vi "CLD1015.vi"() -> ()   [LabVIEW 2021]
uses:
  <vilib>/Analysis/baseanly.llb/Mean (DBL).vi
  <vilib>/Analysis/NI_AALBase.lvlib
panel:
  in  "Iteration":u64
  in  "Steps":u64
  in  "Stop":dbl
  in  "Start":dbl
  out "Horizontal Pointer Slide":dbl(slide) scale=0.0..100.0
  out "Averaged":cluster{"X":dbl, "Y":dbl}[](graph)
  out "Single shot":cluster{"X":dbl, "Y":dbl}[](graph)
  in  "Set current":bool
  out "Temperature":dbl(graph)
  out "Laser Current":dbl(graph)
  in  "Modulation":bool
  in  "Temperature Unit":i16(ring) caption="Temperature Unit (Degrees Celsius)" items=["Degrees Celsius", "Kelvin", "Degrees Fahrenheit"]
  in  "Disp. Auto-Dim.":bool
  in  "Disp. Brightness":dbl min=0.0 max=1.0 step=0.1
  in  "Send Utility\nSettings":bool
  in  "Send LD/TEC\nSettings":bool
  in  "Temperature Set":dbl=15.0 caption="Temperature" min=15.0 max=45.0 step=0.5
  in  "Laser Current Set":dbl caption="Laser Current" min=0.0 max=0.145 step=0.005
  out "Photodiode Current":dbl caption="Photodiode Current (0)"
  out "Thermopile Voltage":dbl caption="Thermopile Voltage (0)"
  out "Power":dbl caption="Power (0)"
  out "Laser Voltage":dbl caption="Laser Voltage (0)"
  out "Laser Current":dbl
  out "Optical Power Pd":dbl caption="Optical Power Pd (0)"
  out "Optical Power Th":dbl caption="Optical Power Th (0)"
  out "Temperature":dbl
  in  "Turn Off Program":bool
  in  "TEC Switch":bool
  in  "LD Switch":bool
  out "TEC Setpoint High Limit":dbl caption="Setpoint High Limit"
  out "TEC Setpoint Low Limit":dbl caption="Setpoint Low Limit"
  out "TEC Operating Mode":enum16{"Current", "Temperature"}(ring)
  out "LD Current Limit":dbl caption="Laser Diode Current Limit"
  in  "resource name":refnum<visa-resource-name>="Probe_laser"
  # "For the program to work properly one have to connect SAS signal to AI7\n and CLD1015 modulation channel to AO0"
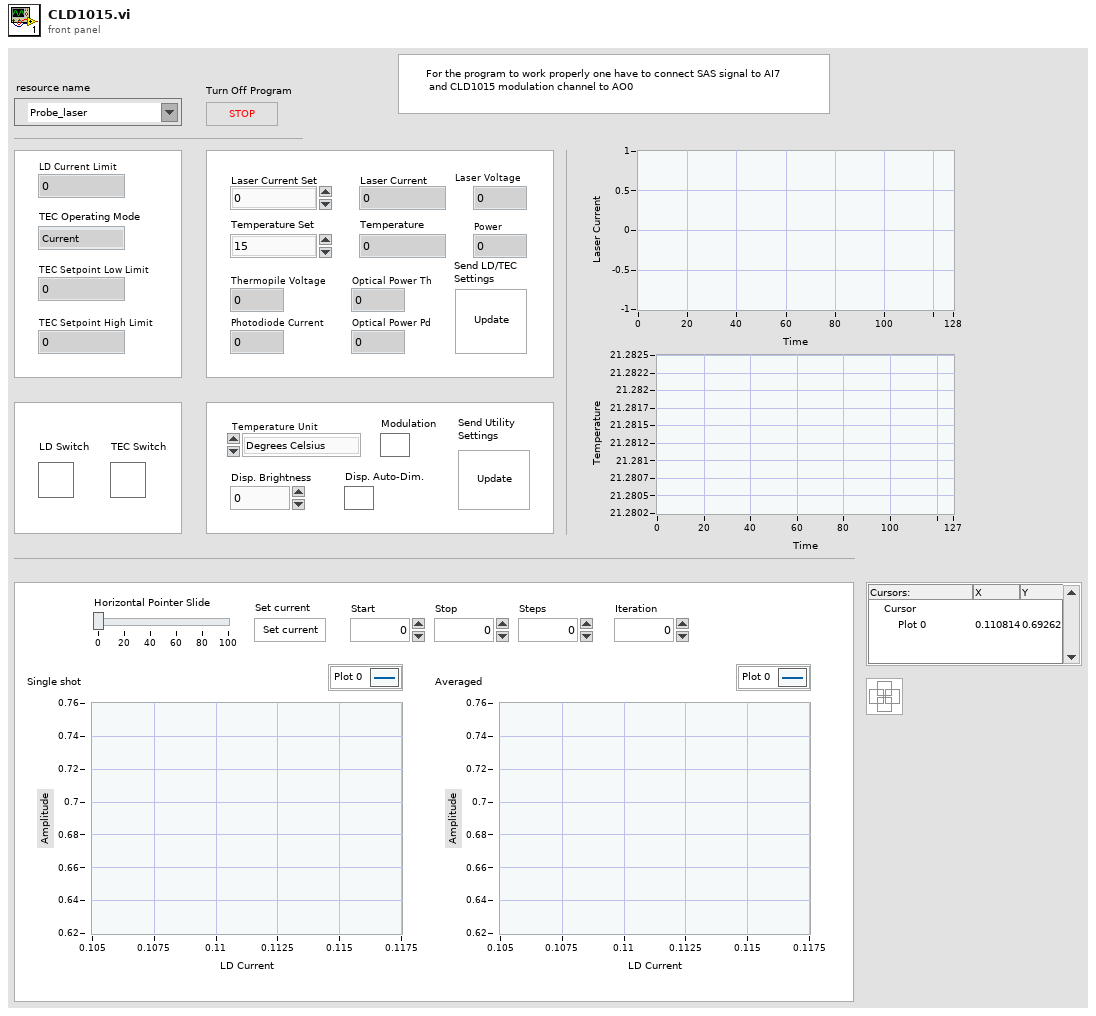
[diagram p1: front panel]
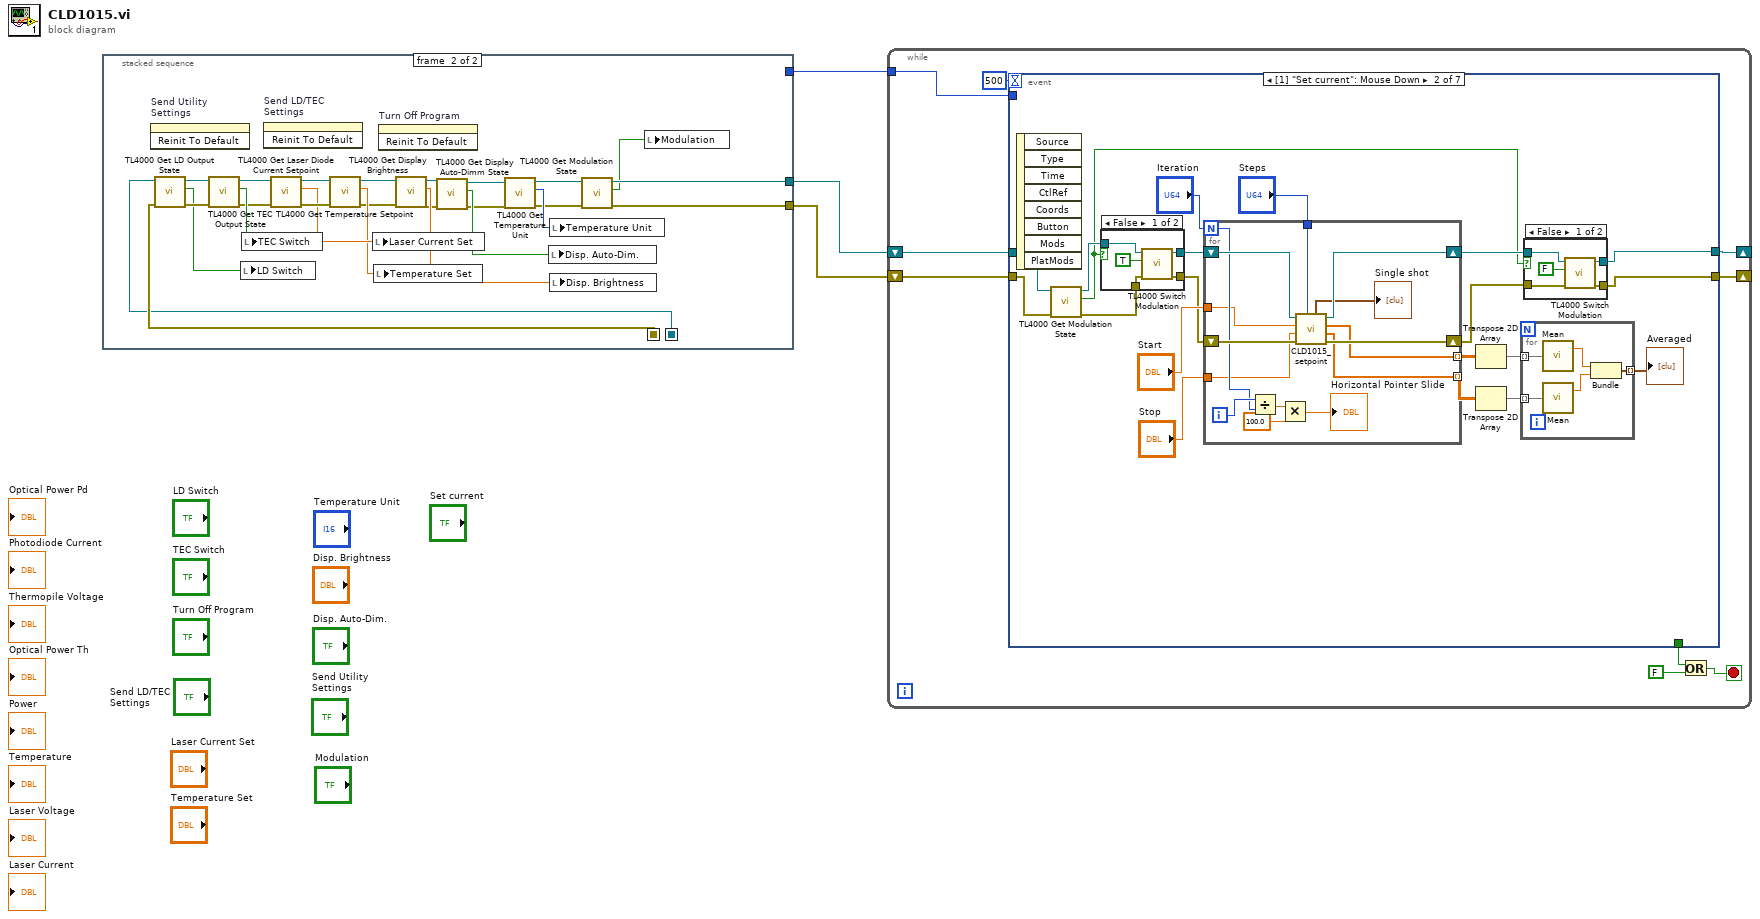
[diagram p0: block diagram]
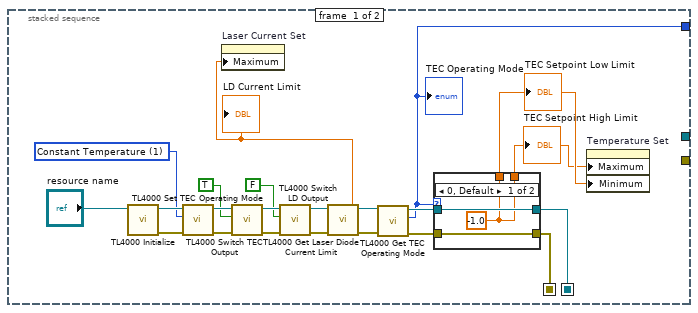
[diagram p2: hidden frame]
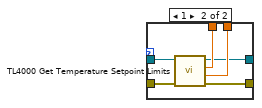
[diagram p3: hidden frame]
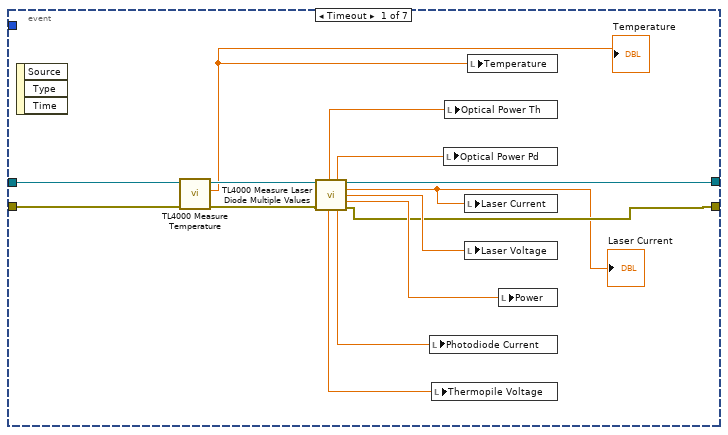
[diagram p4: hidden frame]
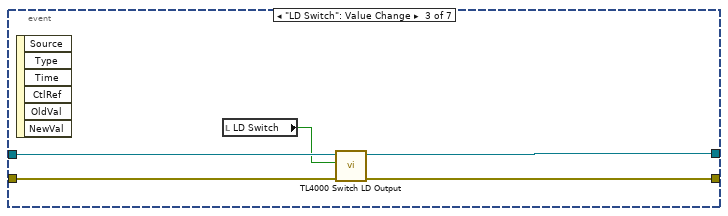
[diagram p7: hidden frame]
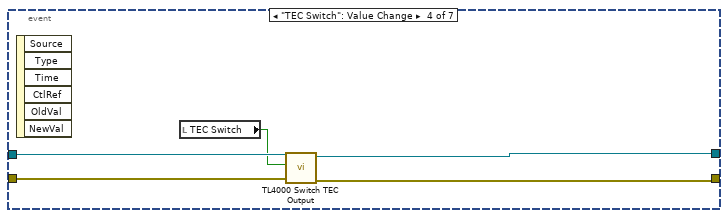
[diagram p8: hidden frame]
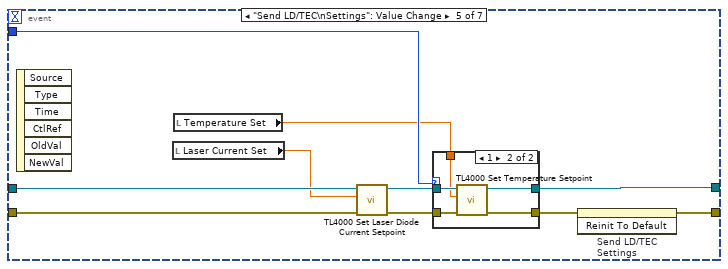
[diagram p9: hidden frame]
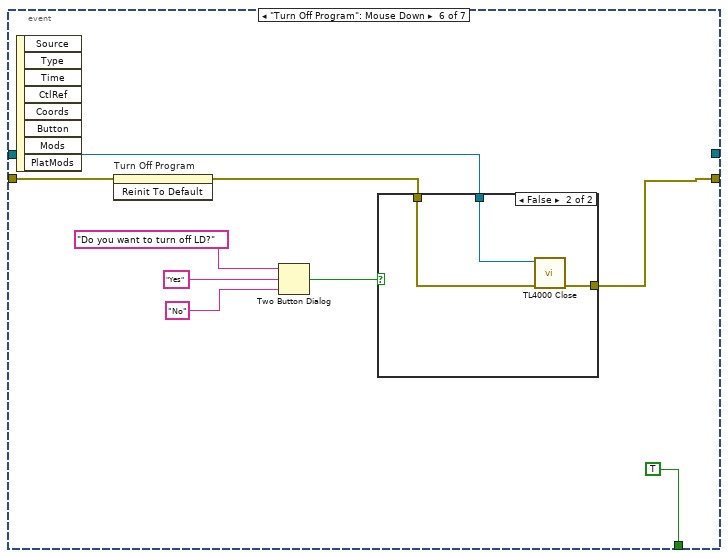
[diagram p11: hidden frame]
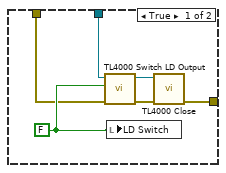
[diagram p12: hidden frame]
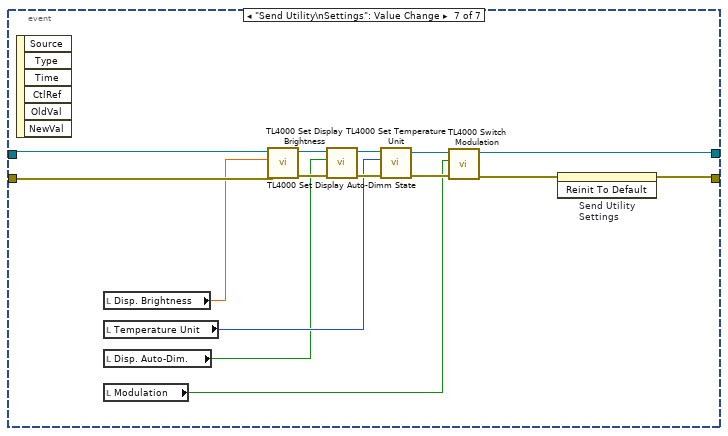
[diagram p13: hidden frame]
diagram:
  n1 = stacked-sequence {
    seq-local: [w9 _] -> [_ w57]
    seq-local: [w8 _] -> [_ w58]
    tunnel: [_ w36] -> w2
    tunnel: [_ w37] -> w1
    tunnel: [w7 _] -> w3
    frame #0 {
      w22 = i16 1 items=["Constant Temperature"=1, "Current Source"=0] ("TEC Operating Mode (Constant Temperature)")
      n2 = call <instrlib>:"TL4000 Initialize.vi"("resource name"="resource name") -> ("error out"=w24:errorcluster, "instrument handle out"=w23:refnum<visa-resource-name>)  [unwired: 9 in]
      n3 = call <instrlib>:"TL4000 Set TEC Operating Mode.vi"("error in (no error)"=w24, "TEC Operating Mode (Constant Temperature)"=w22, "instrument handle"=w23) -> ("error out"=w21:errorcluster, "instrument handle out"=w20:refnum<visa-resource-name>)  [unwired: 7 in]
      n4 = call <instrlib>:"TL4000 Switch TEC Output.vi"("error in (no error)"=w21, "TEC Output (Off)"=TRUE, "instrument handle"=w20) -> ("error out"=w18:errorcluster, "instrument handle out"=w17:refnum<visa-resource-name>)  [unwired: 7 in]
      n5 = call <instrlib>:"TL4000 Switch LD Output.vi"("error in (no error)"=w18, "LD Output (Off)"=FALSE, "instrument handle"=w17) -> ("error out"=w15:errorcluster, "instrument handle out"=w14:refnum<visa-resource-name>)  [unwired: 7 in]
      n6 = call <instrlib>:"TL4000 Get Laser Diode Current Limit.vi"("error in (no error)"=w15, "instrument handle"=w14) -> ("error out"=w13:errorcluster, "Laser Diode Current Limit"=w6:dbl, "instrument handle out"=w12:refnum<visa-resource-name>)  [unwired: 7 in]
      "LD Current Limit" <- w6
      n7 = property on="Laser Current Set" class="DigNum (strict)"("Maximum"=w6) -> ()  [unwired: 2 in, 2 out]
      n8 = call <instrlib>:"TL4000 Get TEC Operating Mode.vi"("error in (no error)"=w13, "instrument handle"=w12) -> ("error out"=w10:errorcluster, "TEC Operating Mode"=w7:i16, "instrument handle out"=w11:refnum<visa-resource-name>)  [unwired: 7 in]
      "TEC Operating Mode" <- w7
      n9 = case shown="0, Default" w7 {
        tunnel: w11 -> [w28 w33]
        tunnel: w10 -> [w27 w34]
        tunnel: [w26 w32] -> w5
        tunnel: [w26 w31] -> w4
        tunnel: [w28 w30] -> w9
        tunnel: [w27 w29] -> w8
        frame 0, Default {
          w26 = -1.0
        }
        frame 1 {
          n10 = call <instrlib>:"TL4000 Get Temperature Setpoint Limits.vi"("error in (no error)"=w34, "instrument handle"=w33) -> ("error out"=w29:errorcluster, "Setpoint High Limit"=w31:dbl, "Setpoint Low Limit"=w32:dbl, "instrument handle out"=w30:refnum<visa-resource-name>)  [unwired: 6 in]
        }
      }
      "TEC Setpoint Low Limit" <- w5
      "TEC Setpoint High Limit" <- w4
      n11 = property on="Temperature Set" class="DigNum (strict)"("Maximum"=w4, "Minimum"=w5) -> ()  [unwired: 2 in, 2 out]
    }
    frame #1 {
      n12 = invoke on="Send Utility\nSettings" class="Bool (strict)" method="Reinit To Default"() -> ()  [unwired: 3 in, 3 out]
      n13 = call <instrlib>:"TL4000 Get LD Output State.vi"("error in (no error)"=w58, "instrument handle"=w57) -> ("error out"=w59:errorcluster, "LD Output"=w56:bool, "instrument handle out"=w60:refnum<visa-resource-name>)  [unwired: 7 in]
      n14 = call <instrlib>:"TL4000 Get TEC Output State.vi"("error in (no error)"=w59, "instrument handle"=w60) -> ("error out"=w53:errorcluster, "TEC Output"=w55:bool, "instrument handle out"=w54:refnum<visa-resource-name>)  [unwired: 7 in]
      n15 = local write "LD Switch"(w56) -> ()
      n16 = local write "TEC Switch"(w55) -> ()
      n17 = invoke on="Send LD/TEC\nSettings" class="Bool (strict)" method="Reinit To Default"() -> ()  [unwired: 3 in, 3 out]
      n18 = call <instrlib>:"TL4000 Get Laser Diode Current Setpoint.vi"("error in (no error)"=w53, "instrument handle"=w54) -> ("error out"=w51:errorcluster, "Laser Diode Current Setpoint"=w50:dbl, "instrument handle out"=w52:refnum<visa-resource-name>)  [unwired: 7 in]
      n19 = call <instrlib>:"TL4000 Get Temperature Setpoint.vi"("error in (no error)"=w51, "instrument handle"=w52) -> ("error out"=w40:errorcluster, "Temperature Setpoint"=w49:dbl, "instrument handle out"=w41:refnum<visa-resource-name>)  [unwired: 7 in]
      n20 = local write "Laser Current Set"(w50) -> ()
      n21 = local write "Temperature Set"(w49) -> ()
      n22 = invoke on="Turn Off Program" class="Bool" method="Reinit To Default"() -> ()  [unwired: 3 in, 3 out]
      n23 = call <instrlib>:"TL4000 Get Display Brightness.vi"("error in (no error)"=w40, "instrument handle"=w41) -> ("error out"=w45:errorcluster, "Brightness"=w46:dbl, "instrument handle out"=w42:refnum<visa-resource-name>)  [unwired: 7 in]
      n24 = call <instrlib>:"TL4000 Get Display Auto-Dimm State.vi"("error in (no error)"=w45, "instrument handle"=w42) -> ("error out"=w44:errorcluster, "Auto-Dimm State"=w47:bool, "instrument handle out"=w43:refnum<visa-resource-name>)  [unwired: 7 in]
      n25 = call <instrlib>:"TL4000 Get Temperature Unit.vi"("error in (no error)"=w44, "instrument handle"=w43) -> ("error out"=w38:errorcluster, "Temperature Unit"=w48:i16, "instrument handle out"=w39:refnum<visa-resource-name>)  [unwired: 7 in]
      n26 = local write "Disp. Auto-Dim."(w47) -> ()
      n27 = local write "Temperature Unit"(w48) -> ()
      n28 = local write "Disp. Brightness"(w46) -> ()
      n29 = call <instrlib>:"TL4000 Get Modulation State.vi"("error in (no error)"=w38, "instrument handle"=w39) -> ("error out"=w37:errorcluster, "Modulation State"=w35:bool, "instrument handle out"=w36:refnum<visa-resource-name>)  [unwired: 7 in]
      n30 = local write "Modulation"(w35) -> ()
    }
  }
  n31 = while {
    shift-right: [w68] -> _
    shift-left: w1 -> [w69]
    tunnel: w3 -> [w62]
    shift-right: [w67] -> _
    shift-left: w2 -> [w61]
    stop <- w66 stop-if-true
    n32 = event shown="[1] \"Set current\": Mouse Down" {
      selector: _ -> [_ _ _ _ _ _ _]
      dyn-events: _ -> [_ _ _ _ _ _ _]
      timeout: 500 -> [_ _ _ _ _ _ _]
      tunnel: w61 -> [w83 w94 w142 w147 w157 w166 w193]
      tunnel: w69 -> [w82 w93 w141 w146 w148 w172 w192]
      tunnel: [w72 w85 w139 w144 w149 w165 w188] -> w68
      tunnel: [w73 w86 w138 w145 w151 _ w185] -> w67
      tunnel: [_ _ _ _ _ TRUE _] -> w64
      tunnel: w62 -> [_ _ _ _ w155 _ _]
      event Timeout {
        n33 = event-data() -> ()  [unwired: 1 in, 3 out]
        n34 = call <instrlib>:"TL4000 Measure Temperature.vi"("error in (no error)"=w82, "instrument handle"=w83) -> ("error out"=w80:errorcluster, "Temperature"=w71:dbl, "instrument handle out"=w81:refnum<visa-resource-name>)  [unwired: 7 in]
        "Temperature" <- w71
        n35 = call <instrlib>:"TL4000 Measure Laser Diode Multiple Values.vi"("instrument handle"=w81, "error in (no error)"=w80) -> ("Optical Power Th (0)"=w79:dbl, "Optical Power Pd (0)"=w78:dbl, "instrument handle out"=w73:refnum<visa-resource-name>, "Laser Current"=w70:dbl, "Laser Voltage (0)"=w77:dbl, "Power (0)"=w76:dbl, "Thermopile Voltage (0)"=w75:dbl, "Photodiode Current (0)"=w74:dbl, "error out"=w72:errorcluster)  [unwired: 5 in]
        "Laser Current" <- w70
        n36 = local write "Photodiode Current"(w74) -> ()
        n37 = local write "Thermopile Voltage"(w75) -> ()
        n38 = local write "Optical Power Pd"(w78) -> ()
        n39 = local write "Optical Power Th"(w79) -> ()
        n40 = local write "Laser Current"(w70) -> ()
        n41 = local write "Laser Voltage"(w77) -> ()
        n42 = local write "Temperature"(w71) -> ()
        n43 = local write "Power"(w76) -> ()
      }
      event "Set current": Mouse Down {
        n44 = event-data() -> ()  [unwired: 1 in, 8 out]
        n45 = call <instrlib>:"TL4000 Get Modulation State.vi"("error in (no error)"=w93, "instrument handle"=w94) -> ("error out"=w90:errorcluster, "Modulation State"=w84:bool, "instrument handle out"=w91:refnum<visa-resource-name>)  [unwired: 7 in]
        n46 = case shown="False" w84 {
          tunnel: [w114 w117] -> w92
          tunnel: w91 -> [w113 w117]
          tunnel: w90 -> [w112 w116]
          tunnel: [w111 w116] -> w89
          frame False {
            n47 = call <instrlib>:"TL4000 Switch Modulation.vi"("error in (no error)"=w112, "Modulation State (Off)"=TRUE, "instrument handle"=w113) -> ("error out"=w111:errorcluster, "instrument handle out"=w114:refnum<visa-resource-name>)  [unwired: 7 in]
          }
          frame True {
          }
        }
        n48 = for {
          N: "Iteration" -> [w126]
          shift-right: [w135] -> w88
          shift-left: w92 -> [w137]
          shift-right: [w134] -> w87
          shift-left: w89 -> [w136]
          tunnel: [w132] -> w103 mode=indexing
          tunnel: [w131] -> w102 mode=indexing
          tunnel: "Steps" -> [w125]
          tunnel: "Start" -> [w124]
          tunnel: "Stop" -> [w123]
          i -> [w127]
          n49 = Divide(x=w127, y=w126) -> (x/y=w130:dbl)
          n50 = Multiply(x=w130, y=100.0) -> (x*y=→"Horizontal Pointer Slide":dbl)
          n51 = call "CLD1015_setpoint.vi"("steps"=w125, "error CLD1015"=w136, "stop"=w123, "start"=w124, "CLD1015 VISA"=w137) -> ("error out"=w134:errorcluster, "signal"=w132:dbl[], "current"=w131:dbl[], "CLD1015 VISA"=w135:refnum<visa-resource-name>, "XY Graph"=→"Single shot":cluster{"X":dbl, "Y":dbl}[])  [unwired: 2 in]
        }
        n52 = Transpose 2D Array(2D array=w102) -> (transposed array=w101:dbl[][])
        n53 = Transpose 2D Array(2D array=w103) -> (transposed array=w100:dbl[][])
        n54 = for {
          tunnel: w101 -> [w121] mode=indexing
          tunnel: w100 -> [w122] mode=indexing
          tunnel: [w118] -> w99 mode=indexing
          n55 = call-poly <vilib>:"Mean.vi"("X"=w121) -> ("mean"=w120:dbl)  [unwired: 1 out]
          n56 = call-poly <vilib>:"Mean.vi"("X"=w122) -> ("mean"=w119:dbl)  [unwired: 1 out]
          n57 = Bundle("mean"=w120, "mean"=w119) -> (w118:cluster{"mean":dbl, "mean":dbl})  [unwired: 1 in]
        }
        "Averaged" <- w99
        n58 = case shown="False" w84 {
          tunnel: [w107 w110] -> w86
          tunnel: w88 -> [w106 w110]
          tunnel: w87 -> [w105 w109]
          tunnel: [w104 w109] -> w85
          frame False {
            n59 = call <instrlib>:"TL4000 Switch Modulation.vi"("error in (no error)"=w105, "Modulation State (Off)"=FALSE, "instrument handle"=w106) -> ("error out"=w104:errorcluster, "instrument handle out"=w107:refnum<visa-resource-name>)  [unwired: 7 in]
          }
          frame True {
          }
        }
      }
      event "LD Switch": Value Change {
        n60 = event-data() -> ()  [unwired: 1 in, 6 out]
        n61 = local read "LD Switch"() -> (w140:bool)
        n62 = call <instrlib>:"TL4000 Switch LD Output.vi"("error in (no error)"=w141, "LD Output (Off)"=w140, "instrument handle"=w142) -> ("error out"=w139:errorcluster, "instrument handle out"=w138:refnum<visa-resource-name>)  [unwired: 7 in]
      }
      event "TEC Switch": Value Change {
        n63 = event-data() -> ()  [unwired: 1 in, 6 out]
        n64 = local read "TEC Switch"() -> (w143:bool)
        n65 = call <instrlib>:"TL4000 Switch TEC Output.vi"("error in (no error)"=w146, "TEC Output (Off)"=w143, "instrument handle"=w147) -> ("error out"=w144:errorcluster, "instrument handle out"=w145:refnum<visa-resource-name>)  [unwired: 7 in]
      }
      event "Send LD/TEC\nSettings": Value Change {
        n66 = event-data() -> ()  [unwired: 1 in, 6 out]
        n67 = local read "Laser Current Set"() -> (w156:dbl)
        n68 = local read "Temperature Set"() -> (w152:dbl)
        n69 = call <instrlib>:"TL4000 Set Laser Diode Current Setpoint.vi"("error in (no error)"=w148, "Laser Diode Current Setpoint (0.0)"=w156, "instrument handle"=w157) -> ("error out"=w153:errorcluster, "instrument handle out"=w154:refnum<visa-resource-name>)  [unwired: 7 in]
        n70 = case shown="1" w155 {
          tunnel: w154 -> [w159 w162]
          tunnel: w153 -> [w158 w164]
          tunnel: [w159 w161] -> w151
          tunnel: [w158 w163] -> w150
          tunnel: w152 -> [_ w160]
          frame 0, Default {
          }
          frame 1 {
            n71 = call <instrlib>:"TL4000 Set Temperature Setpoint.vi"("error in (no error)"=w164, "Temperature Setpoint (25.0)"=w160, "instrument handle"=w162) -> ("error out"=w163:errorcluster, "instrument handle out"=w161:refnum<visa-resource-name>)  [unwired: 7 in]
          }
        }
        n72 = invoke on="Send LD/TEC\nSettings" class="Bool (strict)" method="Reinit To Default"(error in=w150) -> (error out=w149:errorcluster)  [unwired: 2 in, 2 out]
      }
      event "Turn Off Program": Mouse Down {
        n73 = event-data() -> ()  [unwired: 1 in, 8 out]
        n74 = invoke on="Turn Off Program" class="Bool" method="Reinit To Default"(error in=w172) -> (error out=w167:errorcluster)  [unwired: 2 in, 2 out]
        n75 = Two Button Dialog(message="Do you want to turn off LD?", 1:"No" ("F button name (\"Cancel\")"), 2:"Yes" ("T button name (\"OK\")")) -> (T button?=w168:bool)
        n76 = case shown="False" w168 {
          tunnel: w167 -> [w178 w180]
          tunnel: w166 -> [w177 w181]
          tunnel: [w174 w182] -> w165
          frame True {
            w179 = FALSE
            n77 = call <instrlib>:"TL4000 Switch LD Output.vi"("error in (no error)"=w178, "LD Output (Off)"=w179, "instrument handle"=w177) -> ("error out"=w175:errorcluster, "instrument handle out"=w176:refnum<visa-resource-name>)  [unwired: 7 in]
            n78 = local write "LD Switch"(w179) -> ()
            n79 = call <instrlib>:"TL4000 Close.vi"("error in (no error)"=w175, "instrument handle"=w176) -> ("error out"=w174:errorcluster)  [unwired: 9 in]
          }
          frame False {
            n80 = call <instrlib>:"TL4000 Close.vi"("error in (no error)"=w180, "instrument handle"=w181) -> ("error out"=w182:errorcluster)  [unwired: 9 in]
          }
        }
      }
      event "Send Utility\nSettings": Value Change {
        n81 = event-data() -> ()  [unwired: 1 in, 6 out]
        n82 = local read "Disp. Brightness"() -> (w189:dbl)
        n83 = local read "Temperature Unit"() -> (w191:i16)
        n84 = local read "Disp. Auto-Dim."() -> (w190:bool)
        n85 = local read "Modulation"() -> (w183:bool)
        n86 = call <instrlib>:"TL4000 Set Display Brightness.vi"("error in (no error)"=w192, "Brightness (1.0)"=w189, "instrument handle"=w193) -> ("error out"=w197:errorcluster, "instrument handle out"=w196:refnum<visa-resource-name>)  [unwired: 7 in]
        n87 = call <instrlib>:"TL4000 Set Display Auto-Dimm State.vi"("error in (no error)"=w197, "Auto-Dimm (Disable)"=w190, "instrument handle"=w196) -> ("error out"=w195:errorcluster, "instrument handle out"=w194:refnum<visa-resource-name>)  [unwired: 7 in]
        n88 = call <instrlib>:"TL4000 Set Temperature Unit.vi"("error in (no error)"=w195, "Temperature Unit (Degrees Celsius)"=w191, "instrument handle"=w194) -> ("error out"=w187:errorcluster, "instrument handle out"=w186:refnum<visa-resource-name>)  [unwired: 7 in]
        n89 = call <instrlib>:"TL4000 Switch Modulation.vi"("error in (no error)"=w187, "Modulation State (Off)"=w183, "instrument handle"=w186) -> ("error out"=w184:errorcluster, "instrument handle out"=w185:refnum<visa-resource-name>)  [unwired: 7 in]
        n90 = invoke on="Send Utility\nSettings" class="Bool (strict)" method="Reinit To Default"(error in=w184) -> (error out=w188:errorcluster)  [unwired: 2 in, 2 out]
      }
    }
    n91 = Or(x=w64, y=FALSE) -> (x .or. y?=w66:bool)
  }
